vi "create map range.vi"(8 "error in (no error)":errorcluster, 11 "map range":T1) -> (0 "error out":errorcluster, 3 "<JSON> map range":string)   [LabVIEW 2019]
uses:
  <vilib>/JDP Science/JSONtext/support/Format JSON Object.vi
  <vilib>/JDP Science/JSONtext/JSONtext.lvlib
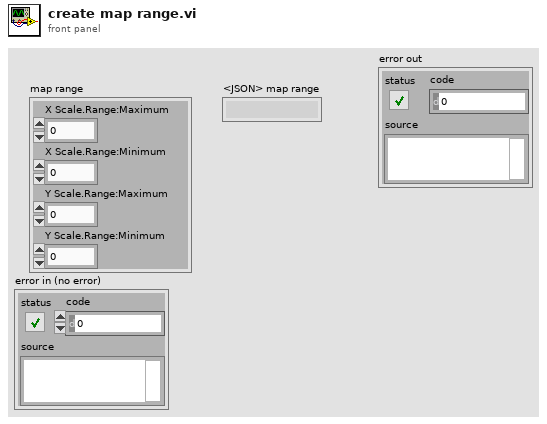
[diagram p1: front panel]
types:
  T1 = cluster{"X Scale.Range:Maximum":dbl, "X Scale.Range:Minimum":dbl, "Y Scale.Range:Maximum":dbl, "Y Scale.Range:Minimum":dbl}
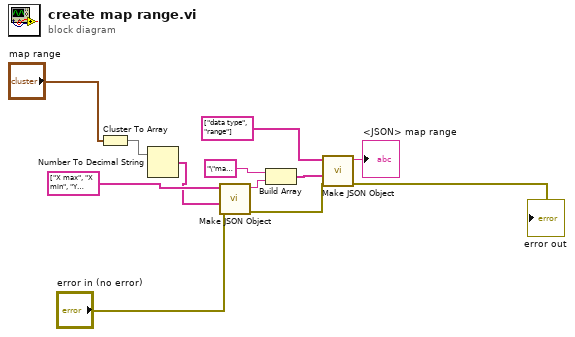
[diagram p0: block diagram]
diagram:
  n1 = Cluster To Array(cluster="map range") -> (array=w5:dbl[])
  n2 = Number To Decimal String(number=w5) -> (decimal integer string=w6:string[])  [unwired: 1 in]
  n3 = call <vilib>:"Make JSON Object.vi"("error in (no error)"="error in (no error)", "JSON Items"=w6, "Item Names"=string[] ["X max", "X min", "Y max", "Y min"]) -> ("error out"=w3:errorcluster, "<JSON>"=w8:string)  [unwired: 7 in]
  n4 = Build Array("\"map range\"" ("element"), w8) -> (w9:string[])
  n5 = call <vilib>:"Make JSON Object.vi"("error in (no error)"=w3, "JSON Items"=w9, "Item Names"=string[] ["data type", "range"]) -> ("error out"=→"error out":errorcluster, "<JSON>"=→"<JSON> map range":string)  [unwired: 7 in]
